vi "Import Config.vi"(8 "error in (no error)":errorcluster, 10 "JSON Charting Config":T1, 11 "Historian Charting Manager in":refnum<class "Historian Charting Manager.lvclass">) -> (0 "error out":errorcluster, 1 "Plot Groups":string[](array[string]), 2 "Chart Groups":string[](array[string]), 3 "Historian Charting Manager out":refnum<class "Historian Charting Manager.lvclass">)   [LabVIEW 2020, in "VolatusGUI.lvlib" / "Historian Charting Manager.lvclass"]
uses:
  Historian Charting Manager.lvclass
  Historian Charting Manager.lvclass/Historian Charting Manager.ctl
  VolatusGUIElements/VolatusGUIElements.lvlib
  Scale.ctl
  X-Axis Type.ctl
  Plot Config.ctl
  Plot Group Config.ctl
  JSON Chart Group.ctl
  VolatusGUI.lvlib
  JSON Plot Config.ctl
  JSON Plot Group.ctl
  JSON Charting Config.ctl
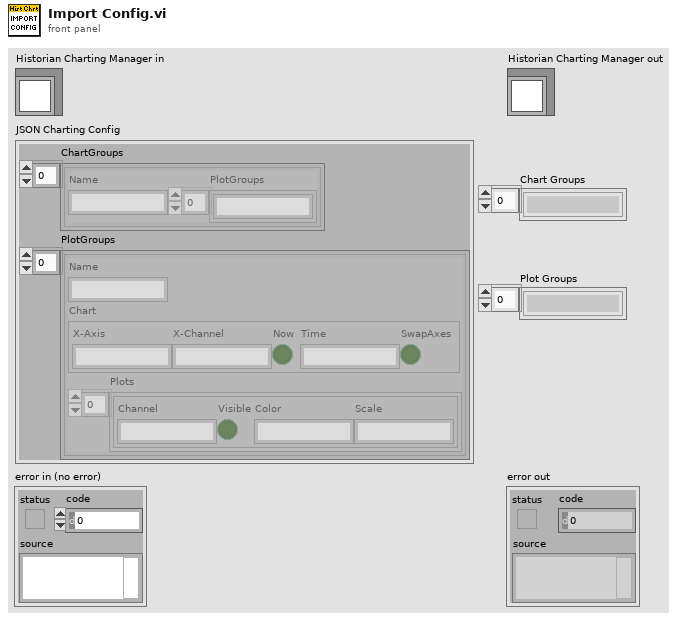
[diagram p1: front panel]
types:
  T1 = typedef "VolatusGUI.lvlib/JSON Charting Config.ctl" = cluster{"ChartGroups":T2[], "PlotGroups":T3[]}
  T2 = typedef "VolatusGUI.lvlib/JSON Chart Group.ctl" = cluster{"Name":string, "PlotGroups":string[]}
  T3 = typedef "VolatusGUI.lvlib/JSON Plot Group.ctl" = cluster{"Name":string, "Chart":cluster{"X-Axis":string, "X-Channel":string, "Now":bool, "Time":string, "SwapAxes":bool}, "Plots":T4[]}
  T4 = typedef "VolatusGUI.lvlib/JSON Plot Config.ctl" = cluster{"Channel":string, "Visible":bool, "Color":string, "Scale":string}
  T5 = typedef "VolatusGUI.lvlib/Historian Charting Manager.lvclass/Plot Group Config.ctl" = cluster{"Name":string, "X-Axis Type":T6, "X-Axis Channel":string, "Plots":T7[], "Lock Now":bool, "Time":string, "Swap Axes":bool}
  T6 = typedef "VolatusGUI.lvlib/Historian Charting Manager.lvclass/X-Axis Type.ctl" = enum16{"Time", "Channel"}
  T7 = typedef "VolatusGUI.lvlib/Historian Charting Manager.lvclass/Plot Config.ctl" = cluster{"Channel":string, "Visible":bool, "Color":u32, "Scale":T8}
  T8 = typedef "VolatusGUI.lvlib/Historian Charting Manager.lvclass/Scale.ctl" = enum16{"Left", "Right"}
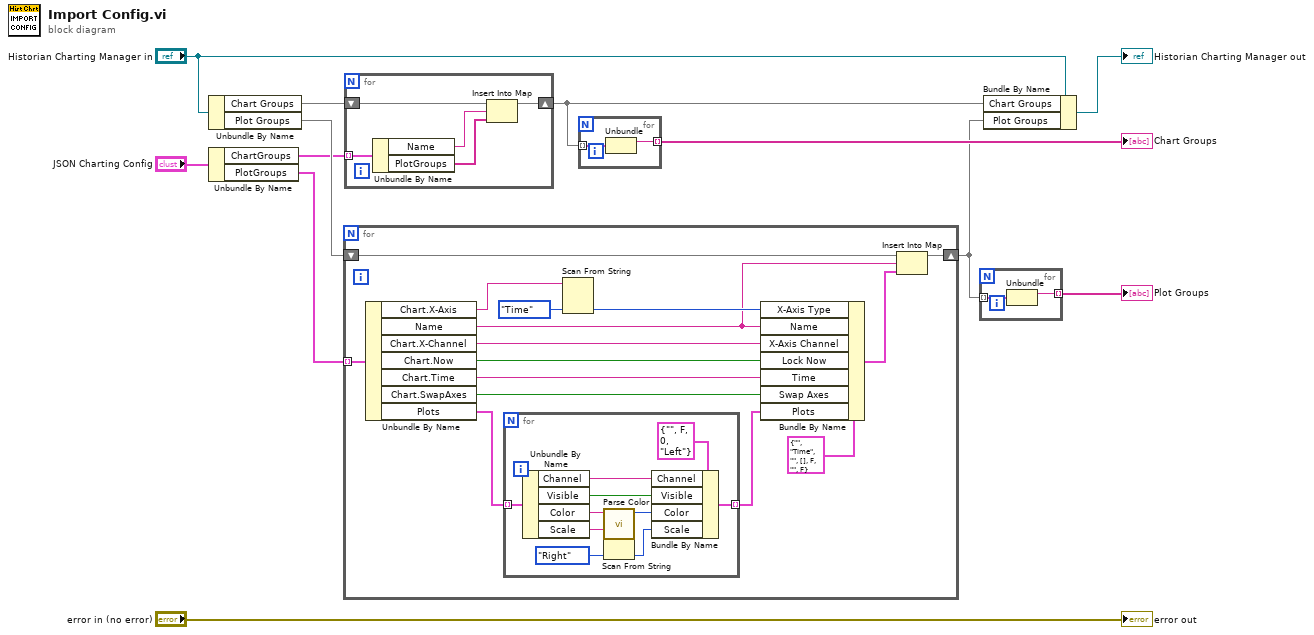
[diagram p0: block diagram]
diagram:
  n1 = Unbundle By Name("Historian Charting Manager in") -> ("Chart Groups"=w6:map{string, string[]}, "Plot Groups"=w8:map{string, T5})
  n2 = Unbundle By Name("JSON Charting Config") -> ("ChartGroups"=w7:T2[], "PlotGroups"=w9:T3[])
  n3 = for {
    tunnel: w9 -> [w27] mode=indexing
    shift-right: [w25] -> w2
    shift-left: w8 -> [w26]
    n4 = Unbundle By Name(w27) -> ("Chart.X-Axis"=w17:string, "Name"=w13:string, "Chart.X-Channel"=w21:string, "Chart.Now"=w22:bool, "Chart.Time"=w20:string, "Chart.SwapAxes"=w19:bool, "Plots"=w24:T4[])
    n5 = for {
      tunnel: w24 -> [w37] mode=indexing
      tunnel: [w28] -> w15 mode=indexing
      n6 = Unbundle By Name(w37) -> ("Channel"=w32:string, "Visible"=w31:bool, "Color"=w36:string, "Scale"=w35:string)
      n7 = call "Parse Color.vi"("Color String"=w36) -> ("Color"=w30:u32)  [unwired: 9 in, 1 out]
      n8 = Scan From String(input string=w35, default 1=Scale."Right" ("Scale")) -> (output 1=w29:T8)  [unwired: 3 in, 3 out]
      n9 = Bundle By Name(cluster=T7 {"Channel"="", "Visible"=FALSE, "Color"=0, "Scale"=enum."Left"} ("Plot Config"), "Channel"=w32, "Visible"=w31, "Color"=w30, "Scale"=w29) -> (w28:T7)
    }
    n10 = Scan From String(input string=w17, default 1=X-Axis_Type."Time" ("X-Axis Type")) -> (output 1=w16:T6)  [unwired: 3 in, 3 out]
    n11 = Bundle By Name(cluster=T5 {"Name"="", "X-Axis Type"=enum."Time", "X-Axis Channel"="", "Plots"=[], "Lock Now"=FALSE, "Time"="", "Swap Axes"=FALSE} ("value"), "X-Axis Type"=w16, "Name"=w13, "X-Axis Channel"=w21, "Lock Now"=w22, "Time"=w20, "Swap Axes"=w19, "Plots"=w15) -> (w14:T5)
    n12 = Insert Into Map(map in=w26, key=w13, value=w14) -> (map out=w25:map{string, T5})  [unwired: 2 out]
  }
  n13 = for {
    tunnel: w7 -> [w42] mode=indexing
    shift-right: [w38] -> w1
    shift-left: w6 -> [w41]
    n14 = Unbundle By Name(w42) -> ("Name"=w39:string, "PlotGroups"=w40:string[])
    n15 = Insert Into Map(map in=w41, key=w39, value=w40) -> (map out=w38:map{string, string[]})  [unwired: 2 out]
  }
  n16 = for {
    tunnel: w1 -> [w44] mode=indexing
    tunnel: [w43] -> w5 mode=indexing
    n17 = Unbundle(w44) -> ("Chart Group"=w43:string)  [unwired: 1 out]
  }
  "Chart Groups" <- w5
  n18 = for {
    tunnel: w2 -> [w46] mode=indexing
    tunnel: [w45] -> w4 mode=indexing
    n19 = Unbundle(w46) -> ("Name"=w45:string)  [unwired: 1 out]
  }
  "Plot Groups" <- w4
  n20 = Bundle By Name(cluster="Historian Charting Manager in", "Chart Groups"=w1, "Plot Groups"=w2) -> (→"Historian Charting Manager out":refnum<class "Historian Charting Manager.lvclass">)
  "error out" <- "error in (no error)"
